vi "readBaseInclinometerSettings.vi"(8 "error in (no error)":errorcluster, 11 "Boot in":refnum<class "Boot.lvclass">) -> (0 "error out":errorcluster, 2 "BaseT7InclinometerSettings":T1, 3 "Boot out":refnum<class "Boot.lvclass">)   [LabVIEW 2016, in "Boot.lvclass"]
uses:
  Boot.lvclass
  DataTypes/Settings/Base/BaseT7InclinometerSettings.ctl
  Boot.lvclass/Boot.ctl
  Settings/Settings/Setting.lvclass
  DataTypes/Settings/M1M3SupportSettings.lvlib
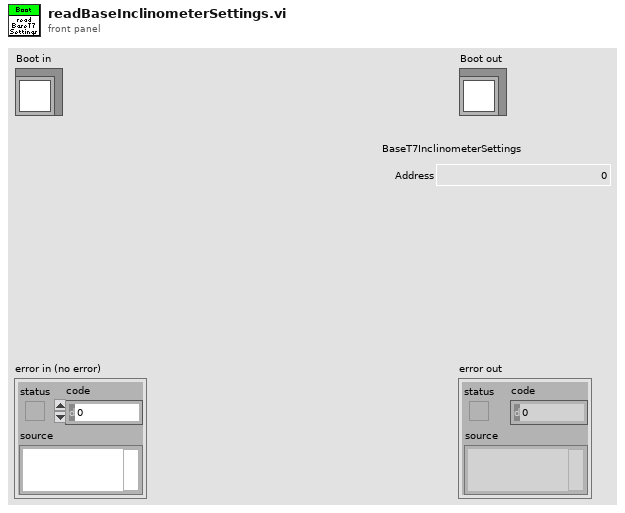
[diagram p1: front panel]
types:
  T1 = typedef "M1M3SupportSettings.lvlib/BaseT7InclinometerSettings.ctl" = cluster{"Address":u8}
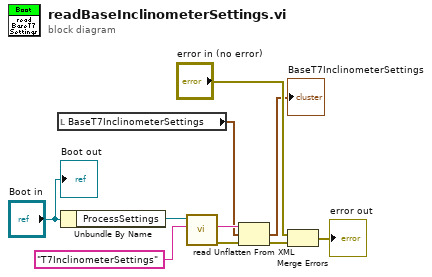
[diagram p0: block diagram]
diagram:
  n1 = local read "BaseT7InclinometerSettings"() -> (w2:T1)
  n2 = Unbundle By Name("Boot in") -> ("ProcessSettings"=w10:refnum<class "Setting.lvclass">)
  n3 = call-dynamic "read.vi"("Name"="T7InclinometerSettings", "BaseSetting in"=w10) -> ("error out"=w6:errorcluster, "XML"=w8:string)  [unwired: 6 in, 2 out]
  n4 = Unflatten From XML(xml string=w8, type=w2, error in (no error)=w6) -> (value=→"BaseT7InclinometerSettings":T1, error out=w3:errorcluster)
  n5 = Merge Errors("error in (no error)", w3) -> (→"error out":errorcluster)
  "Boot out" <- "Boot in"
